vi "Test Priority Queue.vi"(8 "error in":errorcluster, 11 "Test Case In":refnum<class "Messaging Tests.lvclass">) -> (0 "error out":errorcluster, 3 "Test Case Out":refnum<class "Messaging Tests.lvclass">)   [LabVIEW 2020, in "Messaging Tests.lvlib" / "Messaging Tests.lvclass"]
uses:
  Messaging Tests.lvclass
  Messaging Tests.lvclass/Messaging Tests.ctl
  vi.lib/ActorFramework/Stop Msg/Stop Msg.lvclass
  vi.lib/ActorFramework/Message Enqueuer/Message Priority.ctl
  vi.lib/ActorFramework/Message Enqueuer/Message Enqueuer.lvclass
  vi.lib/ActorFramework/Message Queue/Message Queue.lvclass
  vi.lib/ActorFramework/Message Dequeuer/Message Dequeuer.lvclass
  TestActor/Increment Msg/Increment Msg.lvclass
  a81d8e30-c573-480f-ad64-ed782fd7de9b.vi
  <vilib>/Astemes/LUnit/Test Case.lvclass
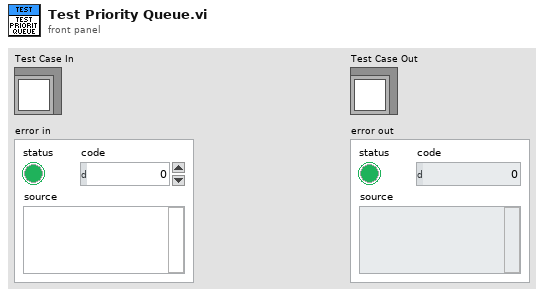
[diagram p1: front panel]
types:
  T1 = typedef "Actor Framework.lvlib/Message Enqueuer.lvclass/Message Priority.ctl" = enum16{"Low", "Normal", "High"}
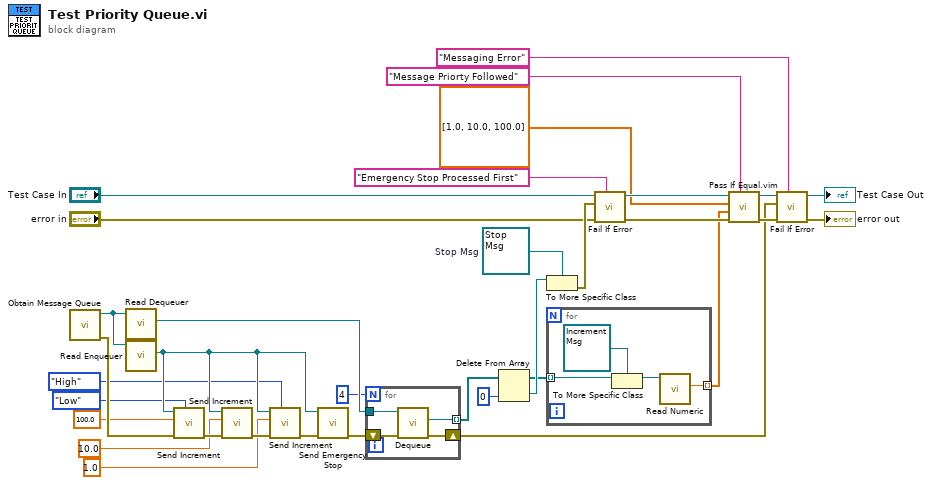
[diagram p0: block diagram]
diagram:
  w16 = refnum<class "Stop Msg.lvclass"> refnum  # Stop Msg
  n1 = call "Obtain Message Queue.vi"() -> ("error out"=w29:errorcluster, "Message Queue"=w12:refnum<class "Message Queue.lvclass">)  [unwired: 10 in]
  n2 = call "Read Dequeuer.vi"("Message Queue"=w12) -> ("Message Dequeuer"=w11:refnum<class "Message Dequeuer.lvclass">)  [unwired: 10 in]
  n3 = call "Read Enqueuer.vi"("Message Queue"=w12) -> ("Message Enqueuer"=w23:refnum<class "Message Enqueuer.lvclass">)  [unwired: 10 in]
  n4 = call "Send Increment.vi"("Message Priority"=Message_Priority."Low", "error in (no error)"=w29, "Numeric"=100.0, "Actor Framework.lvlib:Send Queue"=w23) -> ("error out"=w33:errorcluster)  [unwired: 7 in]
  n5 = call "Send Increment.vi"("error in (no error)"=w33, "Numeric"=10.0, "Actor Framework.lvlib:Send Queue"=w23) -> ("error out"=w32:errorcluster)  [unwired: 8 in]
  n6 = call "Send Increment.vi"("Message Priority"=Message_Priority."High", "error in (no error)"=w32, "Numeric"=1.0, "Actor Framework.lvlib:Send Queue"=w23) -> ("error out"=w31:errorcluster)  [unwired: 7 in]
  n7 = call "Send Emergency Stop.vi"("error in (no error)"=w31, "Message Enqueuer"=w23) -> ("error out"=w30:errorcluster)  [unwired: 9 in]
  n8 = for {
    N: 4 -> [_]
    tunnel: w11 -> [w36]
    tunnel: [w35] -> w19 mode=indexing
    shift-right: [w37] -> w24
    shift-left: w30 -> [w38]
    n9 = call "Dequeue.vi"("error in (no error)"=w38, "Message Dequeuer in"=w36) -> ("error out"=w37:errorcluster, "Message"=w35:refnum<class "Message.lvclass">)  [unwired: 5 in, 3 out]
  }
  n10 = Delete From Array(array=w19, index=0) -> (deleted portion=w17:refnum<class "Message.lvclass">, array with subset deleted=w15:refnum<class "Message.lvclass">[])  [unwired: 1 in]
  n11 = To More Specific Class(target class=w16, reference=w17) -> (error out=w34:errorcluster)  [unwired: 1 in, 1 out]
  n12 = for {
    tunnel: w15 -> [w42] mode=indexing
    tunnel: [w39] -> w6 mode=indexing
    n13 = To More Specific Class(target class=refnum<class "Increment Msg.lvclass"> refnum ("Object"), reference=w42) -> (specific class reference=w40:refnum<class "Increment Msg.lvclass">)  [unwired: 1 in, 1 out]
    n14 = call "Read Numeric.vi"("Increment Msg in"=w40) -> ("Numeric"=w39:dbl)  [unwired: 9 in, 1 out]
  }
  n15 = call <vilib>:"Fail If Error.vi"("Description"="Emergency Stop Processed First", "error in (no error)"="error in", "Assert error"=w34, "LUnit Test Case In"="Test Case In") -> ("error out"=w27:errorcluster, "LUnit Test Case Out"=w9:refnum<class "Messaging Tests.lvclass">)  [unwired: 6 in]
  n16 = call "Pass If Equal.vim"("Description"="Message Priorty Followed", "error in (no error)"=w27, "Actual"=w6, "Expected"=dbl[] [1.0, 10.0, 100.0], "LUnit Test Case In"=w9) -> ("error out"=w25:errorcluster, "LUnit Test Case Out"=w4:refnum<class "Messaging Tests.lvclass">)  [unwired: 5 in]
  n17 = call <vilib>:"Fail If Error.vi"("Description"="Messaging Error", "error in (no error)"=w25, "Assert error"=w24, "LUnit Test Case In"=w4) -> ("error out"=→"error out":errorcluster, "LUnit Test Case Out"=→"Test Case Out":refnum<class "Messaging Tests.lvclass">)  [unwired: 6 in]
